vi "pi_int.vi"(8 "error in":errorcluster, 10 "Interface":u16(ring) items=["RS232", "RS232 DaisyChain", "USB", "USB DaisyChain"]) -> (0 "error out":errorcluster, 1 "Position":dbl[](array[numeric])=[20.8449] format="%.6f", 2 "Identification":string)   [LabVIEW 2014]
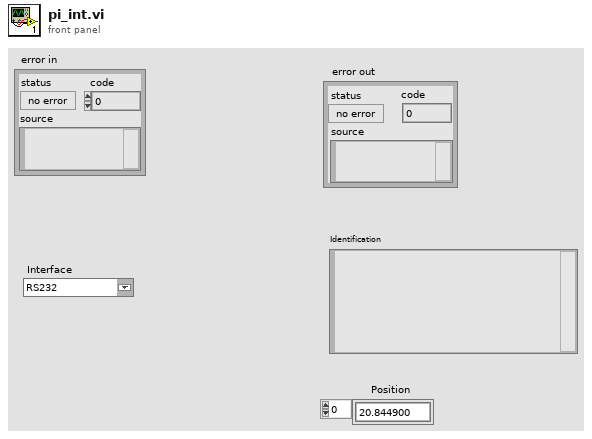
[diagram p1: front panel]
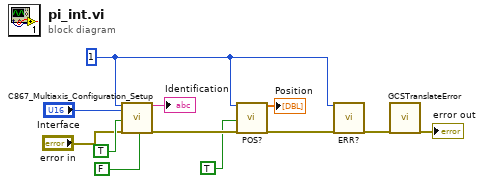
[diagram p0: block diagram]
diagram:
  w6 = 1 ("System no.")
  n1 = call "C867_Multiaxis_Configuration_Setup.vi"("System no."=w6, "Interface"="Interface", "All axes?"=TRUE, "error in"="error in", "Switch servo on?"=FALSE ("Use dialog to define\nconnected stages?")) -> ("Identification"=→"Identification":string, "error out"=w10:errorcluster)  [unwired: 8 in, 5 out]
  n2 = call "POS?.vi"("System no."=w6, "All axes?"=TRUE, "error in"=w10) -> ("Position"=→"Position":dbl[], "error out"=w7:errorcluster)  [unwired: 15 in]
  n3 = call "ERR?.vi"("System no."=w6, "error in"=w7) -> ("error out"=w5:errorcluster)  [unwired: 16 in, 1 out]
  n4 = call "GCSTranslateError.vi"("error in"=w5) -> ("error out"=→"error out":errorcluster)  [unwired: 16 in, 2 out]
